vi "whichLasersForAcq.vi"(3 "LSFM_3 lasers":T2(array[cluster])=[{"Component ID"="405nm", "COM Port"="COM14", "Type "=enum."omicronLuxX", "init"=0}, {"Component ID"="488nm", "COM Port"="COM4", "Type "=enum."omicronLuxX", "init"=0}, {"Component ID"="561nm", "COM Port"="COM27", "Type "=enum."coherentObis", "init"=0}, {"Component ID"="642nm", "COM Port"="COM12", "Type "=enum."omicronLuxX", "init"=0}], 6 "405 nm (aq)":bool=TRUE, 7 "405 nm filter":T3(ring), 8 "488 nm (aq)":bool=TRUE, 9 "488 nm filter":T3(ring)=enum."525/50 [FITC]", 10 "561 nm (aq)":bool=TRUE, 11 "561 nm filter":T3(ring)=enum."605/70 [Cy3]", 12 "642 nm (aq)":bool=TRUE, 13 "642 nm filter":T3(ring)=enum."665/LP [Cy5]") -> (16 "Initialized lasers":T2(array[cluster])=[{"Component ID"="561nm", "COM Port"="COM27", "Type "=enum."coherentObis", "init"=0}], 17 "initializedFilters":T1(array[ring])=[enum."460/36 [DAPI]"])   [LabVIEW 2015]
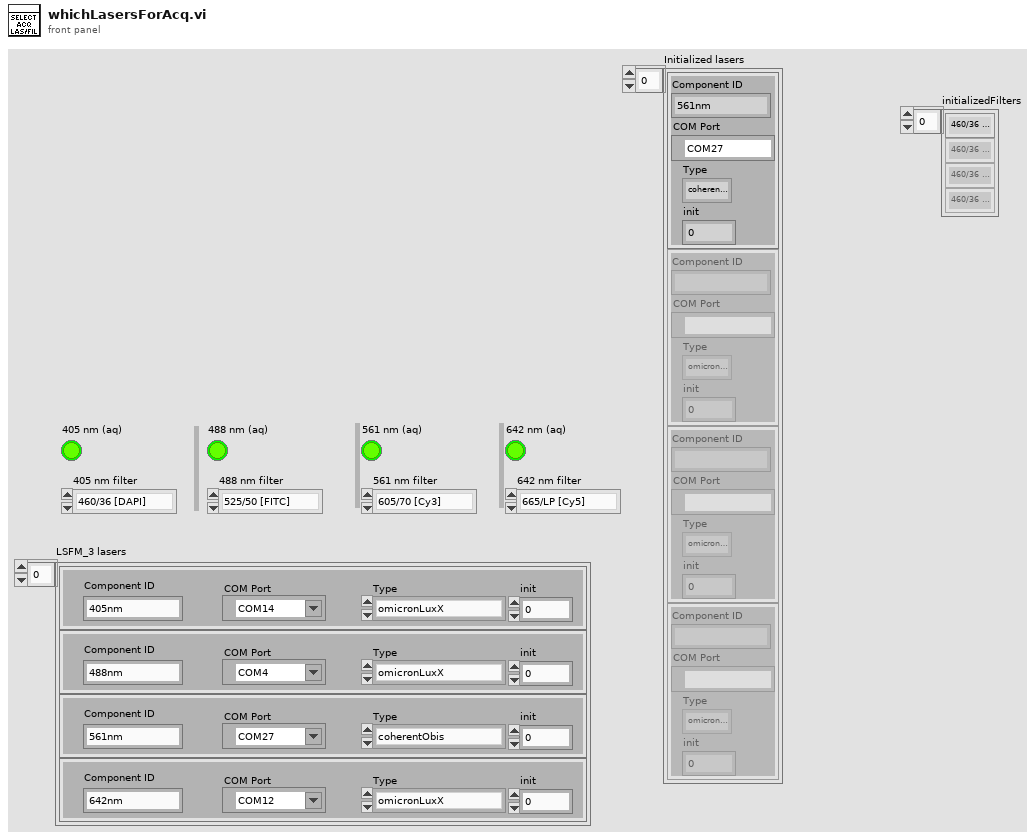
[diagram p1: front panel]
types:
  T1 = enum16{"460/36 [DAPI]", "525/50 [FITC]", "605/70 [Cy3]", "665/LP [Cy5]", "Empty-1", "Empty-2"}[]
  T2 = cluster{"Component ID":string, "COM Port":refnum<visa-resource-name>, "Type ":enum16{"omicronLuxX", "coherentObis"}, "init":i16}[]
  T3 = enum16{"460/36 [DAPI]", "525/50 [FITC]", "605/70 [Cy3]", "665/LP [Cy5]", "Empty-1", "Empty-2"}
  T4 = cluster{"Component ID":string, "COM Port":refnum<visa-resource-name>, "Type ":enum16{"omicronLuxX", "coherentObis"}, "init":i16}
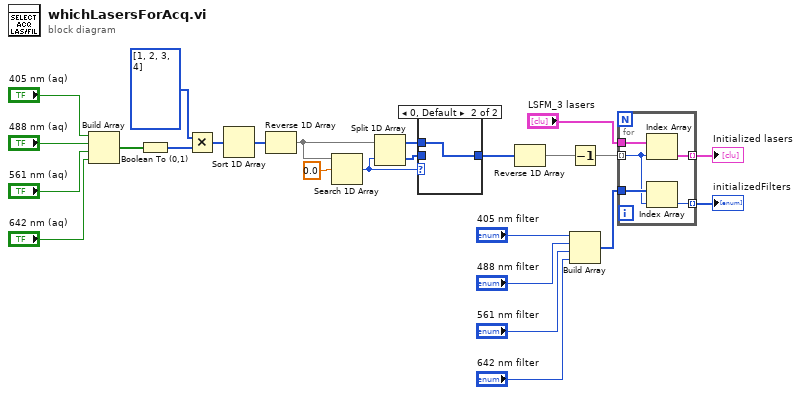
[diagram p0: block diagram]
diagram:
  n1 = Build Array("405 nm (aq)", "488 nm (aq)", "561 nm (aq)", "642 nm (aq)") -> (w1:bool[])
  n2 = Boolean To (0,1)(Boolean=w1) -> (0, 1=w24:i16[])
  n3 = Multiply(x=i16[] [1, 2, 3, 4], y=w24) -> (x*y=w25:i16[])
  n4 = Sort 1D Array(array=w25) -> (sorted array=w18:i16[])
  n5 = Reverse 1D Array(array=w18) -> (reversed array=w20:i16[])
  n6 = Search 1D Array(1D array=w20, element=0.0) -> (index of element=w21:i32)  [unwired: 1 in]
  n7 = Split 1D Array(array=w20, index=w21) -> (first subarray=w22:i16[], second subarray=w23:i16[])
  n8 = case shown="0, Default" w21 {
    tunnel: w22 -> [_ w27]
    tunnel: w23 -> [w26 _]
    tunnel: [w26 w27] -> w16
    frame -1 {
    }
    frame 0, Default {
    }
  }
  n9 = Reverse 1D Array(array=w16) -> (reversed array=w17:i16[])
  n10 = Decrement(x=w17) -> (x-1=w14:i16[])
  n11 = Build Array("405 nm filter", "488 nm filter", "561 nm filter", "642 nm filter") -> (w9:T1)
  n12 = for {
    tunnel: w14 -> [w29] mode=indexing
    tunnel: "LSFM_3 lasers" -> [w32]
    tunnel: [w31] -> w8 mode=indexing
    tunnel: w9 -> [w30]
    tunnel: [w28] -> w7 mode=indexing
    n13 = Index Array(array=w32, index=w29) -> (element=w31:T4)
    n14 = Index Array(array=w30, index=w29) -> (element=w28:T3)
  }
  "Initialized lasers" <- w8
  "initializedFilters" <- w7
